vi "FP_SubVI.vi"(0 "High Byte":u8, 3 "Low Byte":u8) -> (7 "Fuel Pressure":u16)   [LabVIEW 2012]
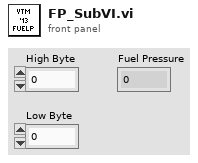
[diagram p1: front panel]
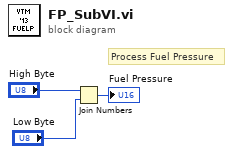
[diagram p0: block diagram]
diagram:
  # "Process Fuel Pressure"
  n1 = Join Numbers(hi="High Byte", lo="Low Byte") -> ((hi.lo)=→"Fuel Pressure":u16)
